vi "PLL_PID.vi"(8 "error in (no error)":errorcluster, 9 "Oscillator []":waveform(dbl), 10 "Target []":waveform(dbl), 11 "LockinDAQ in":refnum<class "Instrument.DAQ.lvclass">) -> (0 "error out":errorcluster={"status"=TRUE, "code"=-5000, "source"="Input waveform exceeds buffer capacity."}, 1 "phase output (°)":dbl=nan, 2 "frequency output (Hz)":dbl, 3 "LockinDAQ out":refnum<class "Instrument.DAQ.lvclass">)   [LabVIEW 2019, in "Instrument.DAQ.lvclass"]
doc: "Please ensure that at least one period is generated or else the measurement VIs do not work properly."
uses:
  Instrument.DAQ.lvclass
  <vilib>/Waveform/WDTOps.llb/WDT Waveform Duration DBL.vi
  <vilib>/addons/control/pid/pid.llb/PID (DBL).vi
  <vilib>/measure/matone.llb/Extract Single Tone Information 1 Chan.vi
  <vilib>/Analysis/NI_AALPro.lvlib
  <vilib>/addons/control/pid/NI_PID_pid.lvlib
  <vilib>/measure/NI_MAPro.lvlib
  <vilib>/ptbypt/NI_PtbyPt.lvlib
panel:
  out "Phase Chart":cluster{dbl, "output":dbl}(graph)={nan, "output"=nan}
  out "Frequency Chart":T1(graph)
  out "process frequency":dbl format="%.2p"
  out "detected frequency (set point)":dbl format="%.2p"
  in  "PID_Phase":T2={"proportional gain (Kc)"=0.1, "integral time (Ti, min)"=0.0008, "derivative time (Td, min)"=0.0} {"derivative time (Td, min)" format="%.3f"; "integral time (Ti, min)" items=["Take a Coffee"=0.1, "Yawning"=0.01, "Take a Deep Breath"=0.001, "Normal"=0.0008, "A Little Bit Fast"=0.0001, "Fast"=1e-05, "Too Fast"=1e-06]; "proportional gain (Kc)" format="%.3f"}
  in  "PID_Frequency":T2={"proportional gain (Kc)"=0.9, "integral time (Ti, min)"=0.0008, "derivative time (Td, min)"=0.0} {"derivative time (Td, min)" format="%.3f"; "integral time (Ti, min)" items=["Take a Coffee"=0.1, "Yawning"=0.01, "Take a Deep Breath"=0.001, "Normal"=0.0008, "A Little Bit Fast"=0.0001, "Fast"=1e-05, "Too Fast"=1e-06]; "proportional gain (Kc)" format="%.3f"}
  out "Waveform Graph":waveform(dbl)[](graph)=[{"t0"=timestamp(0 s since 1904-01-01), "dt"=1.0, "Y"=[]}, {"t0"=timestamp(0 s since 1904-01-01), "dt"=1.0, "Y"=[]}]
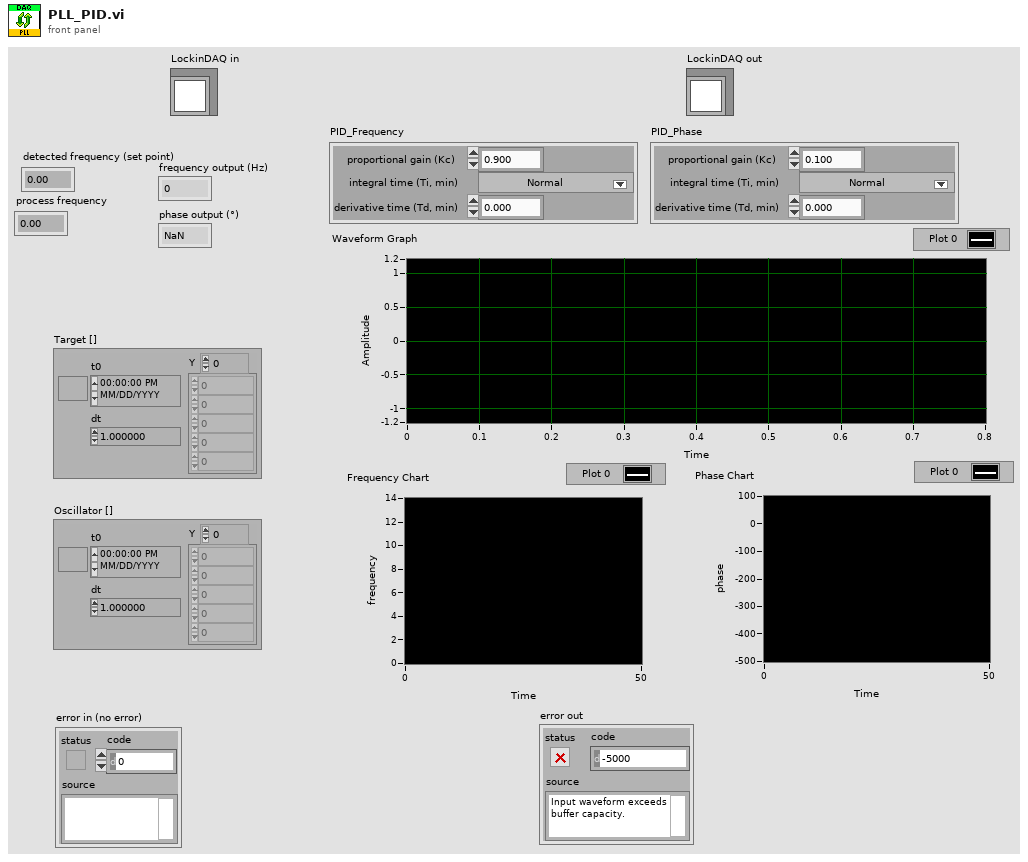
[diagram p1: front panel]
types:
  T1 = cluster{"detected frequency":dbl, "detected frequency":dbl, "output":dbl}
  T2 = cluster{"proportional gain (Kc)":dbl, "integral time (Ti, min)":dbl, "derivative time (Td, min)":dbl}
  T3 = cluster{"detected frequency":dbl, "detected frequency":dbl, "output":dbl}[]
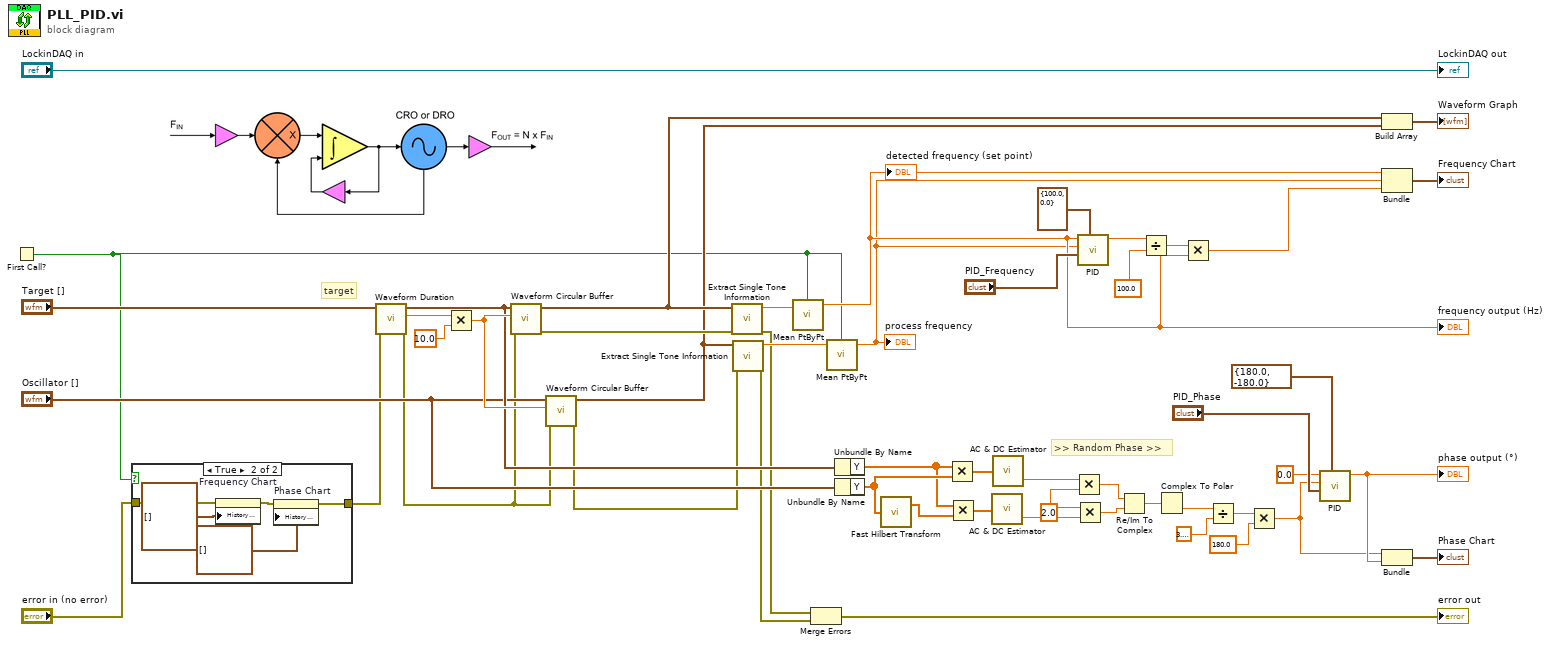
[diagram p0: block diagram]
diagram:
  w36 = 2.0 ("x")
  # "target"
  # ">> Random Phase >>"
  n1 = First Call?() -> (First Call?: T/F=w2:bool)
  n2 = case shown="True" w2 {
    tunnel: [w52 w54] -> w8
    tunnel: "error in (no error)" -> [w52 w53]
    frame False {
    }
    frame True {
      n3 = property on="Frequency Chart" class="WFChart (strict)"(error in=w53, "History Data"=T3 []) -> (error out=w57:errorcluster)  [unwired: 1 in, 1 out]
      n4 = property on="Phase Chart" class="WFChart (strict)"(error in=w57, "History Data"=cluster{dbl, "output":dbl}[] []) -> (error out=w54:errorcluster)  [unwired: 1 in, 1 out]
    }
  }
  n5 = call-poly <vilib>:"Waveform Duration.vi"("error in (no error)"=w8, "waveform in"="Target []") -> ("error out"=w7:errorcluster, "duration"=w31:dbl, "waveform out"=w15:waveform(dbl))  [unwired: 7 in]
  n6 = Multiply(x=w31, y=10.0) -> (x*y=w26:dbl)
  n7 = call "Waveform Circular Buffer.vi"("error in"=w7, "buffer duration (s)"=w26, "waveform in"=w15) -> ("error out"=w28:errorcluster, "waveform out"=w20:waveform(dbl))  [unwired: 7 in]
  n8 = call "Waveform Circular Buffer.vi"("error in"=w7, "buffer duration (s)"=w26, "waveform in"="Oscillator []") -> ("error out"=w5:errorcluster, "waveform out"=w16:waveform(dbl))  [unwired: 7 in]
  n9 = call-poly <vilib>:"Extract Single Tone Information.vi"("error in (no error)"=w28, "time signal in"=w20) -> ("error out"=w11:errorcluster, "detected frequency"=w21:dbl)  [unwired: 4 in, 4 out]
  n10 = call-poly <vilib>:"Extract Single Tone Information.vi"("error in (no error)"=w5, "time signal in"=w16) -> ("error out"=w10:errorcluster, "detected frequency"=w25:dbl)  [unwired: 4 in, 4 out]
  n11 = call <vilib>:"Mean PtByPt.vi"("x"=w21, "initialize"=w2) -> ("mean"=w12:dbl)  [unwired: 2 in, 1 out]
  "frequency output (Hz)" <- w12
  "detected frequency (set point)" <- w12
  n12 = Merge Errors(w11, w10) -> (→"error out":errorcluster)
  n13 = call <vilib>:"Mean PtByPt.vi"("x"=w25, "initialize"=w2) -> ("mean"=w6:dbl)  [unwired: 2 in, 1 out]
  "process frequency" <- w6
  n14 = Unbundle By Name(w15) -> ("Y"=w48:dbl[])
  n15 = Unbundle By Name("Oscillator []") -> ("Y"=w50:dbl[])
  n16 = call <vilib>:"Fast Hilbert Transform.vi"("X"=w50) -> ("Hilbert{X}"=w49:dbl[])  [unwired: 1 out]
  n17 = Multiply(x=w48, y=w50) -> (x*y=w47:dbl[])
  n18 = Multiply(x=w48, y=w49) -> (x*y=w46:dbl[])
  n19 = call <vilib>:"AC & DC Estimator.vi"("Signal (V)"=w46) -> ("DC estimate (V)"=w45:dbl)  [unwired: 1 out]
  n20 = call <vilib>:"AC & DC Estimator.vi"("Signal (V)"=w47) -> ("DC estimate (V)"=w37:dbl)  [unwired: 1 out]
  n21 = Multiply(x=w37, y=w36) -> (x*y=w39:dbl)
  n22 = Multiply(x=w36, y=w45) -> (x*y=w38:dbl)
  n23 = call-poly <vilib>:"PID.vi"("output range"=cluster{"output high":dbl, "output low":dbl} {"output high"=100.0, "output low"=0.0}, "PID gains"="PID_Frequency", "process variable"=w6, "setpoint"=w12) -> ("output"=w22:dbl)  [unwired: 6 in, 1 out]
  n24 = Re/Im To Complex(1:w38, 2:w39) -> (0:w40:cdb)
  n25 = Divide(x=w22, y=100.0) -> (x/y=w23:dbl)
  n26 = Complex To Polar(r * e^(i*theta)=w40) -> (theta=w41:dbl)  [unwired: 1 out]
  n27 = Multiply(x=w23, y=w12) -> (x*y=w13:dbl)
  n28 = Divide(x=w41, y=3.141592653589793) -> (x/y=w43:dbl)
  n29 = Multiply(x=w43, y=180.0) -> (x*y=w4:dbl)
  n30 = call-poly <vilib>:"PID.vi"("output range"=cluster{"output high":dbl, "output low":dbl} {"output high"=180.0, "output low"=-180.0}, "PID gains"="PID_Phase", "process variable"=w4, "setpoint"=0.0) -> ("output"=w18:dbl)  [unwired: 6 in, 1 out]
  "phase output (°)" <- w18
  n31 = Build Array(w20, w16) -> (→"Waveform Graph":waveform(dbl)[])
  n32 = Bundle("mean"=w12, "mean"=w6, w13) -> (→"Frequency Chart":cluster{"mean":dbl, "mean":dbl, dbl})  [unwired: 1 in]
  n33 = Bundle(w4, "output"=w18) -> (→"Phase Chart":cluster{dbl, "output":dbl})  [unwired: 1 in]
  "LockinDAQ out" <- "LockinDAQ in"
